vi "json_call-chain.vi"(7 "indent level":i32, 10 "Call Chain":string[](array[string])) -> (2 "indented string":string)   [LabVIEW 2013, in "Caraya.lvlib" / "Test Result.lvclass"]
uses:
  Test Result.lvclass
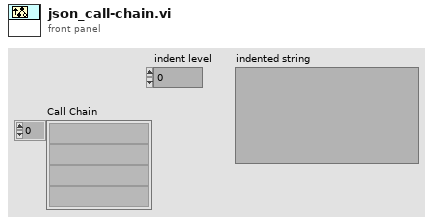
[diagram p1: front panel]
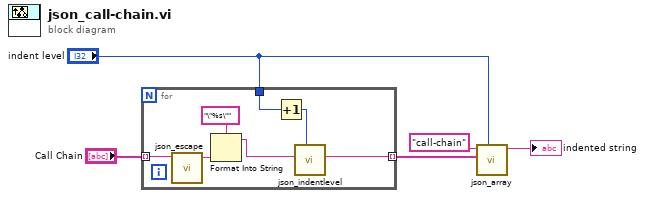
[diagram p0: block diagram]
diagram:
  n1 = for {
    tunnel: "Call Chain" -> [w12] mode=indexing
    tunnel: [w6] -> w2 mode=indexing
    tunnel: "indent level" -> [w8]
    n2 = call "json_escape.vi"("string"=w12) -> ("escaped string"=w10:string)  [unwired: 10 in]
    n3 = Format Into String(format string="\"%s\"", w10) -> (resulting string=w7:string)  [unwired: 2 in, 1 out]
    n4 = Increment(x=w8) -> (x+1=w9:i32)
    n5 = call "json_indentlevel.vi"("indent level"=w9, "string"=w7) -> ("indented string"=w6:string)  [unwired: 9 in]
  }
  n6 = call "json_array.vi"("indent level"="indent level", "Array of JSON Elements"=w2, "name"="call-chain" ("string")) -> ("indented string"=→"indented string":string)  [unwired: 8 in]
